vi "Loop_ACT_Wrist.vi"() -> ()   [LabVIEW 2017, in "Arm.lvlib"]
uses:
  Arm.lvlib
  _SHARE ALL/TypeDef Share All/CLUSTER_TalonOutput.ctl
  _SHARE ALL/TypeDef Share All/CLUSTER_TalonInput.ctl
  System Drivers/Phoenix-LabVIEW/Motor Controller/Controls/CTRE_Phoenix_MotorControl_ControlMode.ctl
  TypeDef/CLUSTER_PID.ctl
  _SHARE ALL/TypeDef Share All/CONTROL_PositonGraph.ctl
  Globals/Global_Device_IDs.vi
  _SHARE ALL/Global Share All/Global_STOP.vi
  Global_SM Write_Data Out.vi
  System Drivers/Phoenix-LabVIEW/Motor Controller/Get/CTRE_Phoenix_MotorController_GetSelectedSensorData.vi
  System Drivers/Phoenix-LabVIEW/Motor Controller/Get/CTRE_Phoenix_MotorController_GetVoltage.vi
  Global_ACT Write_Data Out.vi
  <vilib>/Rock Robotics/WPI/RobotDrive/WPI_RobotDriveOpen2MotorWithExistingMotors.vi
panel:
  in  "Display Graph":bool
  out "Position Closed Loop Plots":T1
  out "Wrist Input":T2 {"Talon Mode" items=["PercentOutput"=0, "Position"=1, "Velocity"=2, "Current"=3, "Follower"=5, "MotionProfile"=6, "MotionMagic"=7, "MotionMagicArc"=8, "MotionProfileArc"=10, "Disabled"=15]}
  out "Wrist Output":T5
  out "Cycle Time (S)":dbl format="%.3g"
  in  "Target Time(ms)":u32=50
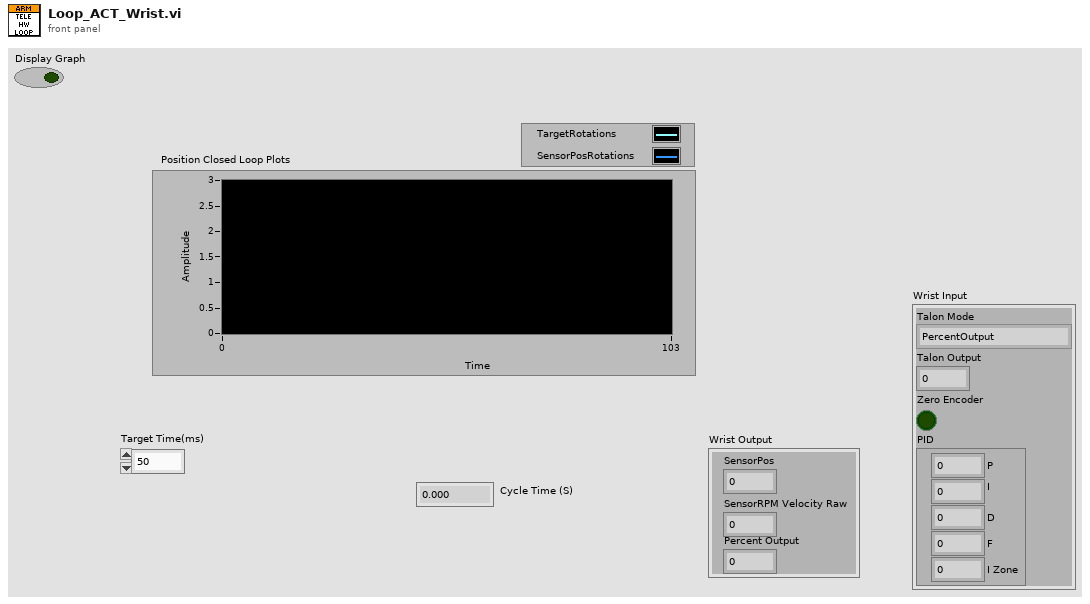
[diagram p1: front panel]
types:
  T1 = typedef "CONTROL_PositonGraph.ctl" = cluster{dbl, "Position (Raw Sensor Units)":i32}
  T2 = typedef "CLUSTER_TalonInput.ctl" = cluster{"Talon Mode":T3, "Talon Output":dbl, "Zero Encoder":bool, "PID":T4}
  T3 = typedef "CTRE_Phoenix_MotorControl_ControlMode.ctl" = u16
  T4 = typedef "CLUSTER_PID.ctl" = cluster{"P":dbl, "I":dbl, "D":dbl, "F":dbl, "I Zone":dbl}
  T5 = typedef "CLUSTER_TalonOutput.ctl" = cluster{"SensorPos":i32, "SensorRPM Velocity Raw":i32, "Percent Output":dbl}
  T6 = typedef "CLUSTER_Arm_Device_IDs.ctl" = cluster{"Elbow Setup":T7, "Telescope Setup":T7, "Wrist Setup":T7}
  T7 = typedef "CLUSTER_Talon_Setup.ctl" = cluster{"Talon SRX ID":u8, "PhaseSensor":bool, "Invert Motor?":bool, "Phoenix Feedback Select":T8, "pidLoopldx":i32, "PID":T4}
  T8 = typedef "CTRE_Phoenix_MotorControl_FeedbackDevice.ctl" = i8
  T9 = typedef "WPI_MotorControlDeviceRef.ctl" = cluster{"DeviceStatus":errorcluster, "Type":T10, "PWM":cluster{"PWM Channel":T11, "DeadBand":T12}, "CAN":cluster{"Device Number":u8, "SetOutput VI Ref":variant, "GetOutput VI Ref":variant, "Enable VI Ref":variant, "Disable VI Ref":variant, "Data":variant}, "Invert":bool, "DIO PWM":cluster{"PWM \"Enable\" Channel":T11, "DIOChannel":T13, "PWM Rate":dbl}}
  T10 = typedef "WPI_MotorControlType.ctl" = enum16{"PWM", "CAN", "DIO PWM"}
  T11 = typedef "FPGA_DIOPWMChannel.ctl" = enum8{"PWM 0", "PWM 1", "PWM 2", "PWM 3", "PWM 4", "PWM 5", "PWM 6", "PWM 7", "PWM 8", "PWM 9", "PWM MXP 0", "PWM MXP 1", "PWM MXP 2", "PWM MXP 3", "PWM MXP 4", "PWM MXP 5", "PWM MXP 6", "PWM MXP 7", "PWM MXP 8", "PWM MXP 9", "Invalid"}
  T12 = typedef "WPI_PWMDeadband.ctl" = cluster{"Name":string, "maxPositivePwm":i32, "minPositivePwm":i32, "centerPwm":i32, "maxNegativePwm":i32, "minNegativePwm":i32, "angularRange":u16}
  T13 = typedef "FPGA_DIOChannel.ctl" = enum8{"DIO 0", "DIO 1", "DIO 2", "DIO 3", "DIO 4", "DIO 5", "DIO 6", "DIO 7", "DIO 8", "DIO 9", "DIO MXP 0", "DIO MXP 1", "DIO MXP 2", "DIO MXP 3", "DIO MXP 4", "DIO MXP 5", "DIO MXP 6", "DIO MXP 7", "DIO MXP 8", "DIO MXP 9", "DIO MXP 10", "DIO MXP 11", "DIO MXP 12", "DIO MXP 13", "DIO MXP 14", "DIO MXP 15", "SPI Port CS1", "SPI Port CS2", "SPI Port CS3", "SPI Port MISO", "SPI Port MOSI", "Invalid"}
  T14 = cluster{"PhoenixMotorControlDevRef":T9, "Wrist Output":T5, "Wrist Input":T2, "Target Time(ms)":u32, "Current Time":timestamp, "Previous Time":timestamp, "Cycle Time (S)":dbl, "Last PID":T4}
  T15 = typedef "WPI_RobotDriveDevRef.ctl" = cluster{"DevStatus":errorcluster, "Motors[]":T9[], "Square Inputs":bool, "Max Output":dbl}
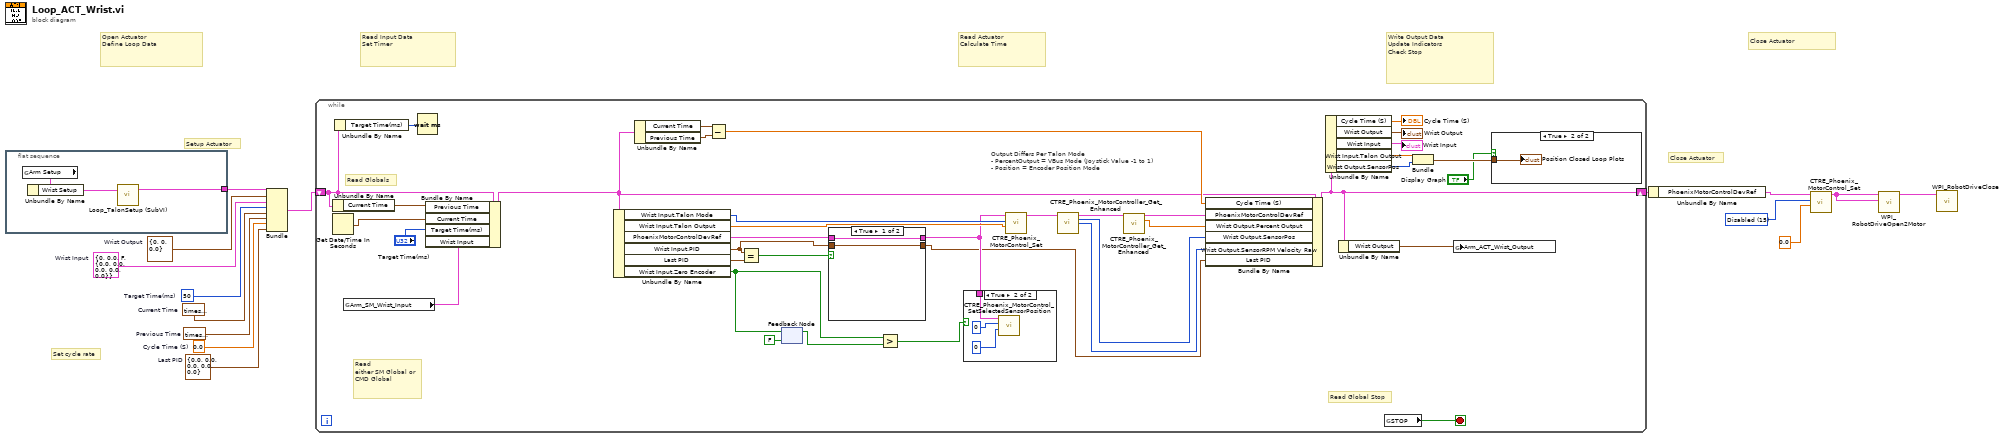
[diagram p0: block diagram]
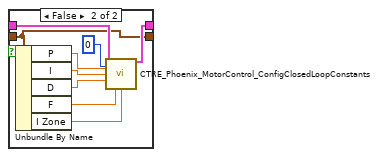
[diagram p2: hidden frame]
diagram:
  w1 = T4 {"P"=0.0, "I"=0.0, "D"=0.0, "F"=0.0, "I Zone"=0.0}  # Last PID
  w5 = T3 15 items=["PercentOutput"=0, "Position"=1, "Velocity"=2, "Current"=3, "Follower"=5, "MotionProfile"=6, "MotionMagic"=7, "MotionMagicArc"=8, "MotionProfileArc"=10, "Disabled"=15] ("Control Mode")
  w7 = T5 {"SensorPos"=0, "SensorRPM Velocity Raw"=0, "Percent Output"=0.0}  # Wrist Output
  w8 = T2 {"Talon Mode"=0, "Talon Output"=0.0, "Zero Encoder"=FALSE, "PID"={"P"=0.0, "I"=0.0, "D"=0.0, "F"=0.0, "I Zone"=0.0}}  # Wrist Input
  w10 = 0.0  # Cycle Time (S)
  w15 = timestamp(0 s since 1904-01-01)  # Previous Time
  w14 = timestamp(0 s since 1904-01-01)  # Current Time
  w13 = u32 50  # Target Time(ms)
  # "Close Actuator"
  # "Write Output Data\nUpdate Indicators\nCheck Stop"
  # "Read Actuator\nCalculate Time"
  # "Read Input Data\nSet Timer"
  # "Open Actuator\nDefine Loop Data"
  # "Set cycle rate"
  # "Close Actuator"
  # "Setup Actuator"
  n1 = flat-sequence {
    tunnel: [w18] -> w9
    frame #0 {
      n2 = global read "Global_Device_IDs.vi" "Arm Setup"() -> (w17:T6)
      n3 = Unbundle By Name(w17) -> ("Wrist Setup"=w16:T7)
      n4 = call "Loop_TalonSetup (SubVI).vi"("Elbow Setup"=w16) -> ("PhoenixMotorControlDevRef"=w18:T9)  [unwired: 10 in]
    }
  }
  n5 = Bundle("PhoenixMotorControlDevRef"=w9, "Wrist Output"=w7, "Wrist Input"=w8, "Target Time(ms)"=w13, "Current Time"=w14, "Previous Time"=w15, "Cycle Time (S)"=w10, "Last PID"=w1) -> (w12:T14)  [unwired: 1 in]
  n6 = while {
    shift-right: [w48] -> w11
    shift-left: w12 -> [w50]
    stop <- w56 stop-if-true
    # "Output Differs Per Talon Mode\n- PercentOutput = VBus Mode (Joystick Value -1 to 1)\n- Position = Encoder Position Mode"
    # "Read\neither SM Global or CMD Global"
    # "Read Globals"
    # "Read Global Stop"
    n7 = Unbundle By Name(w50) -> ("Current Time"=w54:timestamp)
    n8 = Get Date/Time In Seconds() -> (seconds since 1Jan1904=w55:timestamp)
    n9 = Unbundle By Name(w50) -> ("Target Time(ms)"=w49:u32)
    n10 = global read "Global_SM Write_Data Out.vi" "Arm_SM_Wrist_Input"() -> (w44:T2)
    n11 = Wait (ms)(milliseconds to wait=w49) -> ()  [unwired: 1 out]
    n12 = Bundle By Name(cluster=w50, "Previous Time"=w54, "Current Time"=w55, "Target Time(ms)"="Target Time(ms)", "Wrist Input"=w44) -> (w30:T14)
    n13 = Unbundle By Name(w30) -> ("Wrist Input.Talon Mode"=w43:T3, "Wrist Input.Talon Output"=w42:dbl, "PhoenixMotorControlDevRef"=w29:T9, "Wrist Input.PID"=w25:T4, "Last PID"=w26:T4, "Wrist Input.Zero Encoder"=w20:bool)
    n14 = Unbundle By Name(w30) -> ("Current Time"=w53:timestamp, "Previous Time"=w52:timestamp)
    n15 = Subtract(x=w53, y=w52) -> (x-y=w46:dbl)
    n16 = Equal?(x=w25, y=w26) -> (x = y?=w23:bool)
    n17 = feedback #1(FALSE) -> (w21:bool)
    n18 = feedback-in #1(w20) -> ()
    n19 = case shown="True" w23 {
      tunnel: w29 -> [w58 w67]
      tunnel: [w58 w66] -> w28
      tunnel: w25 -> [w57 w59]
      tunnel: [w57 w59] -> w24
      frame True {
      }
      frame False {
        n20 = Unbundle By Name(w59) -> ("P"=w64:dbl, "I"=w63:dbl, "D"=w62:dbl, "F"=w61:dbl, "I Zone"=w60:dbl)
        n21 = call "CTRE_Phoenix_MotorControl_ConfigClosedLoopConstants.vi"("PhoenixMotorControlDevRef"=w67, "slotIdx"=0, "P"=w64, "I"=w63, "D"=w62, "F"=w61, "I Zone"=w60) -> ("PhoenixMotorControlDevRef"=w66:T9)  [unwired: 7 in, 1 out]
      }
    }
    n22 = Greater?(x=w20, y=w21) -> (0:w19:bool)
    n23 = case shown="True" w19 {
      tunnel: w28 -> [_ w71]
      frame False {
      }
      frame True {
        n24 = call "CTRE_Phoenix_MotorControl_SetSelectedSensorPosition.vi"("pidLoopIdx"=u32 0, "New Sensor Position"=0, "PhoenixMotorControlDevRef"=w71) -> ()  [unwired: 7 in, 2 out]
      }
    }
    n25 = call "CTRE_Phoenix_MotorControl_Set.vi"("Output"=w42, "Control Mode"=w43, "PhoenixMotorControlDevRef"=w28) -> ("PhoenixMotorControlDevRef"=w41:T9)  [unwired: 7 in, 1 out]
    n26 = call-poly "CTRE_Phoenix_MotorController_Get_Enhanced.vi"("PhoenixMotorControlDevRef"=w41) -> ("PhoenixMotorControlDevRef"=w40:T9, "Position (Raw Sensor Units)"=w36:i32, "Velocity (Raw Sensor Units per 100 ms)"=w37:i32)  [unwired: 11 in, 1 out]
    n27 = call-poly "CTRE_Phoenix_MotorController_Get_Enhanced.vi"("PhoenixMotorControlDevRef"=w40) -> ("PhoenixMotorControlDevRef"=w39:T9, "Percent Output"=w38:dbl)  [unwired: 10 in, 3 out]
    n28 = Bundle By Name(cluster=w30, "Cycle Time (S)"=w46, "PhoenixMotorControlDevRef"=w39, "Wrist Output.Percent Output"=w38, "Wrist Output.SensorPos"=w36, "Wrist Output.SensorRPM Velocity Raw"=w37, "Last PID"=w24) -> (w48:T14)
    n29 = Unbundle By Name(w48) -> ("Cycle Time (S)"=→"Cycle Time (S)":dbl, "Wrist Output"=→"Wrist Output":T5, "Wrist Input"=→"Wrist Input":T2, "Wrist Input.Talon Output"=w33:dbl, "Wrist Output.SensorPos"=w32:i32)
    n30 = Unbundle By Name(w48) -> ("Wrist Output"=w45:T5)
    n31 = global read "Global_STOP.vi" "STOP"() -> (w56:bool)
    n32 = Bundle("Talon Output"=w33, "SensorPos"=w32) -> (w31:cluster{"Talon Output":dbl, "SensorPos":i32})  [unwired: 1 in]
    n33 = global write "Global_ACT Write_Data Out.vi" "Arm_ACT_Wrist_Output"(w45) -> ()
    n34 = case shown="True" "Display Graph" {
      tunnel: w31 -> [_ w68]
      frame False {
      }
      frame True {
        "Position Closed Loop Plots" <- w68
      }
    }
  }
  n35 = Unbundle By Name(w11) -> ("PhoenixMotorControlDevRef"=w6:T9)
  n36 = call "CTRE_Phoenix_MotorControl_Set.vi"("Output"=0.0, "Control Mode"=w5, "PhoenixMotorControlDevRef"=w6) -> ("PhoenixMotorControlDevRef"=w2:T9)  [unwired: 7 in, 1 out]
  n37 = call-poly <vilib>:"WPI_RobotDriveOpen2Motor.vi"("Right Motor Dev Ref"=w2, "Left Motor Dev Ref"=w2) -> ("RobotDriveDevRef"=w4:T15)  [unwired: 8 in, 1 out]
  n38 = call <vilib>:"WPI_RobotDriveClose.vi"("RobotDriveDevRef"=w4) -> ()  [unwired: 10 in, 1 out]
